vi "Firmware Manager.vi"(5 "Firmware Backup Folder":path, 6 "cRIO IP Address":string="172.16.0.2", 7 "Action":u8(ring) items=["Back Up Firmware to Files", "Update Firmware from Files"]) -> ()   [LabVIEW 2018]
doc: "Utility to save/restore/copy LabVIEW RT target configurations.\nUsage:\n rtcp [-c|-d] [-s] source destination\nwhere source, destination can be either IP address or folder path\nOptions: \ndefault (no option) - copy from target to target (using host's temporary folder):\n rtcp IPsource IPdestination\n-c - save an image of RT system in local folder:\n rtcp -c IPsource dst_folder\n-d - apply saved image or a patch to target:\n rtcp -d src_folder IPdestination\n-s - copy software only, skipping all other files (Installed Software Checkbox)"
uses:
  <vilib>/Utility/config.llb/Read Key (String).vi
  <vilib>/Utility/config.llb/NI_LVConfig.lvlib
panel:
  in  "Browse IP":bool
  out "Description":string
  in  "Exit":bool
  in  "Start Copying":bool
  out "Messages":string
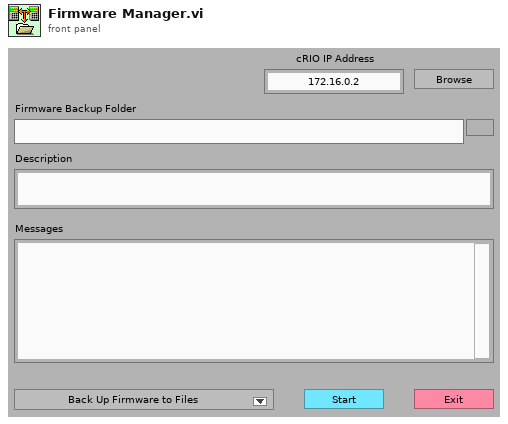
[diagram p1: front panel]
types:
  T1 = cluster{"Model":string, "MAC Address":string, "Hostname":string}
  T2 = typedef "NI_LVConfig.lvlib/Config Data RefNum.ctl" = refnum<k1>
  T3 = cluster{"cRIO IP Address":string, string, "Firmware Backup Folder":path, "Source":enum32{"RT Target", "Folder"}}
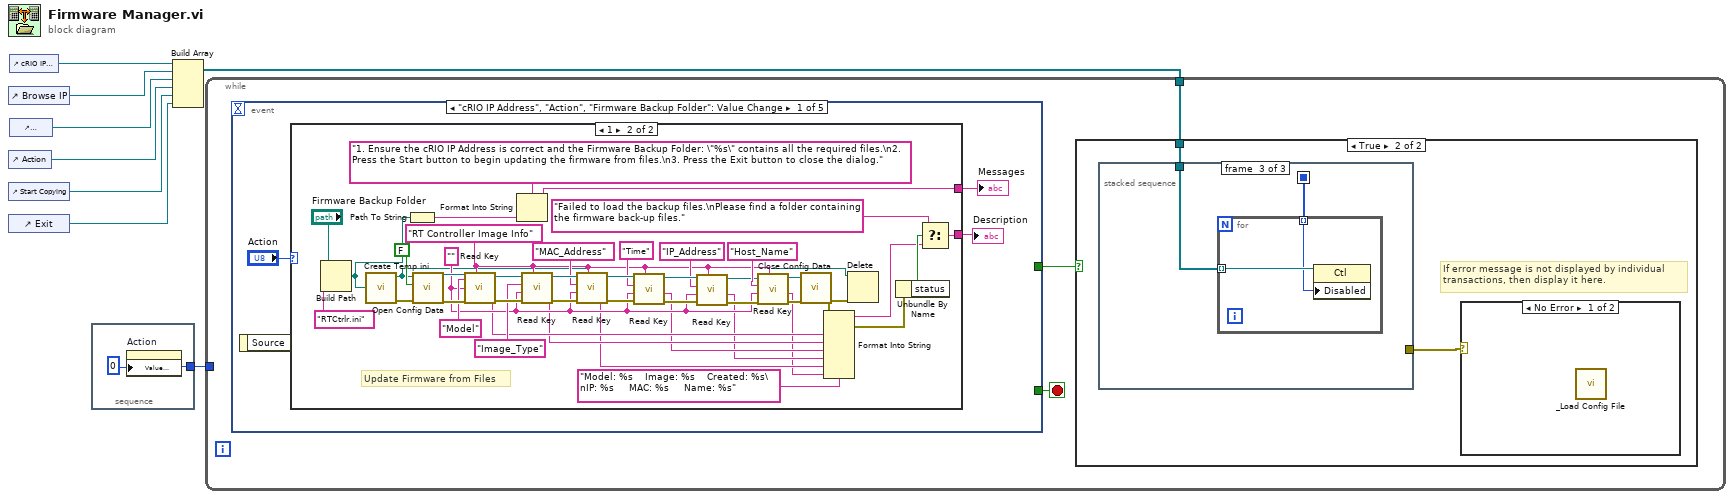
[diagram p0: block diagram]
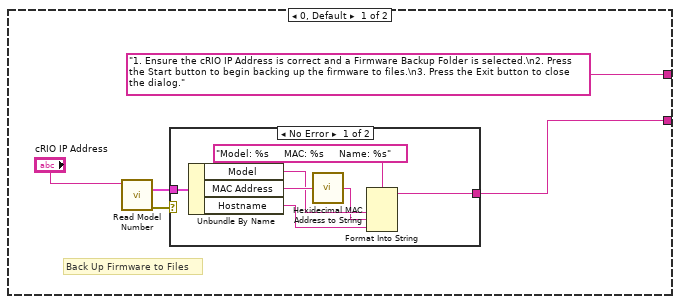
[diagram p2: hidden frame]
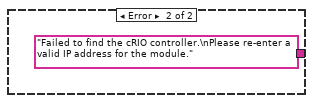
[diagram p3: hidden frame]
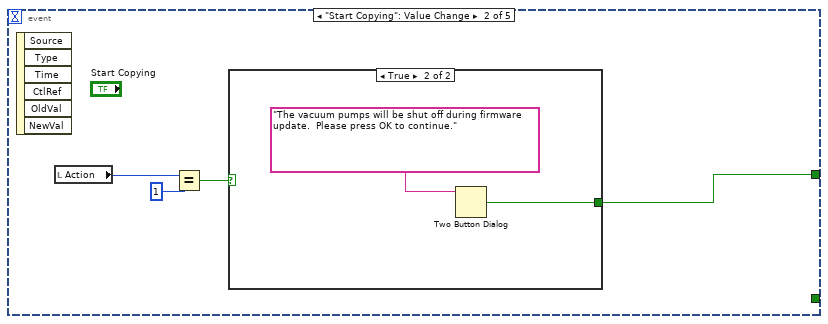
[diagram p4: hidden frame]
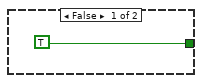
[diagram p5: hidden frame]
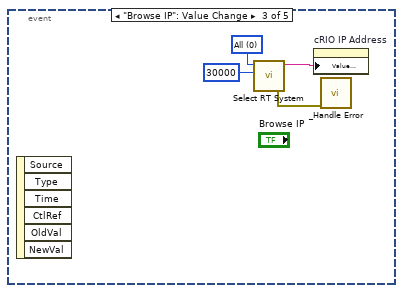
[diagram p6: hidden frame]
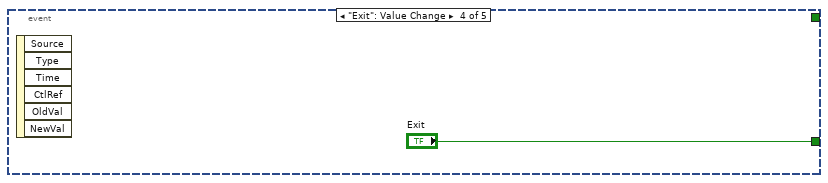
[diagram p7: hidden frame]
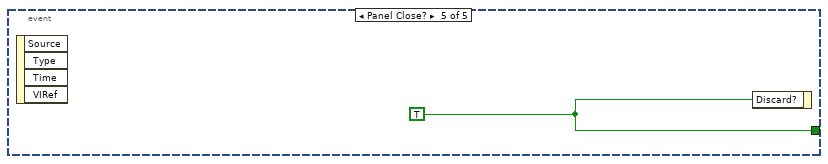
[diagram p8: hidden frame]
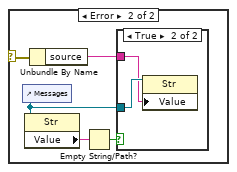
[diagram p10: hidden frame]
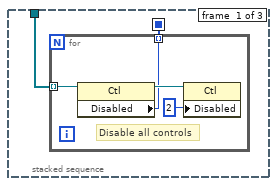
[diagram p12: hidden frame]
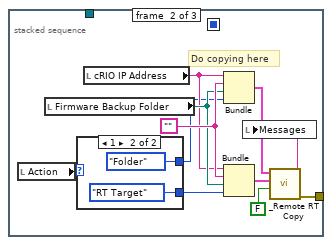
[diagram p13: hidden frame]
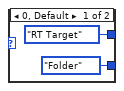
[diagram p14: hidden frame]
diagram:
  n1 = control-ref of="Browse IP"() -> (w7:refnum<vi>)
  n2 = control-ref of="Action"() -> (w5:refnum<vi>)
  n3 = control-ref of="Start Copying"() -> (w3:refnum<vi>)
  n4 = control-ref of="Exit"() -> (w2:refnum<vi>)
  n5 = control-ref of="cRIO IP Address"() -> (w8:refnum<vi>)
  n6 = control-ref of="Firmware Backup Folder"() -> (w6:refnum<vi>)
  n7 = stacked-sequence {
    tunnel: [w9] -> w1
    frame #0 {
      w9 = u8 0
      n8 = property on="Action" class="Ring (strict)"("Value (Signaling)"=w9) -> ()  [unwired: 2 in, 2 out]
    }
  }
  n9 = Build Array(w8, w7, w6, w5, w3, w2) -> (w4:refnum<vi>[])
  n10 = while {
    tunnel: w4 -> [w10]
    tunnel: w1 -> [_]
    stop <- w11 stop-if-true
    n11 = event shown="[0] \"cRIO IP Address\", \"Action\", \"Firmware Backup Folder\": Value Change" {
      selector: _ -> [_ _ _ _ _]
      dyn-events: _ -> [_ _ _ _ _]
      timeout: _ -> [_ _ _ _ _]
      tunnel: [_ _ _ "Exit" w85] -> w11
      tunnel: [_ w73 _ _ _] -> w12
      event "cRIO IP Address", "Action", "Firmware Backup Folder": Value Change {
        n12 = event-data() -> ()  [unwired: 2 out]
        n13 = case shown="1" "Action" {
          tunnel: [w18 w38] -> w15
          tunnel: ["1. Ensure the cRIO IP Address is correct and a Firmware Backup Folder is selected.\n2. Press the Start button to begin backing up the firmware to files.\n3. Press the Exit button to close the dialog." ("t") w34] -> w13
          frame 0, Default {
            # "Back Up Firmware to Files"
            n14 = call "Read Model Number.vi"("String"="cRIO IP Address") -> ("error out"=w19:errorcluster, "Target Info"=w20:T1)  [unwired: 9 in]
            n15 = case shown="No Error" w19 {
              tunnel: w20 -> [w27 _]
              tunnel: [w21 "Failed to find the cRIO controller.\nPlease re-enter a valid IP address for the module." ("t")] -> w18
              frame No Error {
                n16 = Unbundle By Name(w27) -> ("Model"=w24:string, "MAC Address"=w26:string, "Hostname"=w22:string)
                n17 = call <userlib>:"Hexidecimal MAC Address to String.vi"("MAC Address"=w26) -> ("MAC Address ("=w23:string)
                n18 = Format Into String(format string="Model: %s     MAC: %s     Name: %s", w24, w23, w22) -> (resulting string=w21:string)  [unwired: 2 in, 1 out]
              }
              frame Error {
              }
            }
          }
          frame 1 {
            w47 = ""
            w36 = "RT Controller Image Info" ("section")
            # "Update Firmware from Files"
            n19 = Build Path(base path="Firmware Backup Folder", name or relative path="RTCtrlr.ini") -> (appended path=w32:path)
            n20 = call "Create Temp ini.vi"("Original ini path"=w32) -> ("error out"=w31:errorcluster, "Temp ini path"=w29:path)  [unwired: 9 in]
            n21 = Path To String(path=w32) -> (string=w35:string)
            n22 = call <vilib>:"Open Config Data.vi"("error in (no error)"=w31, "create file if necessary (T)"=FALSE ("create file if necessary? (T)"), "configuration file path"=w29) -> ("error out"=w70:errorcluster, "refnum"=w71:T2)  [unwired: 6 in, 1 out]
            n23 = call-poly <vilib>:"Read Key.vi"("section"=w36, "error in (no error)"=w70, "default value"=w47, "key"="Model", "refnum"=w71) -> ("error out"=w67:errorcluster, "value"=w45:string, "refnum out"=w68:T2)  [unwired: 1 in, 3 out]
            n24 = Format Into String(format string="1. Ensure the cRIO IP Address is correct and the Firmware Backup Folder: \"%s\" contains all the required files.\n2. Press the Start button to begin updating the firmware from files.\n3. Press the Exit button to close the dialog." ("t"), w35) -> (resulting string=w34:string)  [unwired: 2 in, 1 out]
            n25 = call-poly <vilib>:"Read Key.vi"("section"=w36, "error in (no error)"=w67, "default value"=w47, "key"="Image_Type", "refnum"=w68) -> ("error out"=w64:errorcluster, "value"=w44:string, "refnum out"=w65:T2)  [unwired: 1 in, 3 out]
            n26 = call-poly <vilib>:"Read Key.vi"("section"=w36, "error in (no error)"=w64, "default value"=w47, "key"="MAC_Address", "refnum"=w65) -> ("error out"=w60:errorcluster, "value"=w41:string, "refnum out"=w61:T2)  [unwired: 1 in, 3 out]
            n27 = call-poly <vilib>:"Read Key.vi"("section"=w36, "error in (no error)"=w60, "default value"=w47, "key"="Time", "refnum"=w61) -> ("error out"=w50:errorcluster, "value"=w43:string, "refnum out"=w51:T2)  [unwired: 1 in, 3 out]
            n28 = call-poly <vilib>:"Read Key.vi"("section"=w36, "error in (no error)"=w50, "default value"=w47, "key"="IP_Address", "refnum"=w51) -> ("error out"=w48:errorcluster, "value"=w42:string, "refnum out"=w49:T2)  [unwired: 1 in, 3 out]
            n29 = call-poly <vilib>:"Read Key.vi"("section"=w36, "error in (no error)"=w48, "default value"=w47, "key"="Host_Name", "refnum"=w49) -> ("error out"=w58:errorcluster, "value"=w40:string, "refnum out"=w59:T2)  [unwired: 1 in, 3 out]
            n30 = call <vilib>:"Close Config Data.vi"("error in (no error)"=w58, "refnum"=w59) -> ("error out"=w30:errorcluster)  [unwired: 1 in, 8 out]
            n31 = Format Into String(format string="Model: %s    Image: %s    Created: %s\nIP: %s     MAC: %s     Name: %s", error in=w30, w45, w44, w43, w42, w41, w40) -> (resulting string=w53:string, error out=w55:errorcluster)  [unwired: 1 in]
            n32 = Delete(path (use dialog)=w29, error in=w30) -> ()  [unwired: 3 in, 3 out]
            n33 = Unbundle By Name(w55) -> ("status"=w54:bool)
            n34 = Select(t="Failed to load the backup files.\nPlease find a folder containing the firmware back-up files.", s=w54, f=w53) -> (s? t:f=w38:string)
          }
        }
        "Description" <- w15
        "Messages" <- w13
      }
      event "Start Copying": Value Change {
        n35 = event-data() -> ()  [unwired: 7 out]
        n36 = local read "Action"() -> (w76:u8)
        n37 = Equal?(x=w76, y=u8 1) -> (x = y?=w74:bool)
        n38 = case shown="True" w74 {
          tunnel: [TRUE w78] -> w73
          frame False {
          }
          frame True {
            n39 = Two Button Dialog(message="The vacuum pumps will be shut off during firmware update.  Please press OK to continue.") -> (T button?=w78:bool)  [unwired: 2 out]
          }
        }
      }
      event "Browse IP": Value Change {
        w83 = u16 0 items=["All", "Configured only", "Unconfigured only"] ("Display Mode")
        n40 = event-data() -> ()  [unwired: 7 out]
        n41 = call "Select RT System.vi"("Timeout ms (4000)"=30000, "Display Mode"=w83) -> ("error out"=w80:errorcluster, "IP Addresst Out"=w81:string)  [unwired: 1 in, 3 out]
        n42 = property on="cRIO IP Address" class="Str"("Value (Signaling)"=w81) -> ()  [unwired: 2 in, 2 out]
        n43 = call "_Handle Error.vi"("error in (no error)"=w80) -> ()  [unwired: 2 in, 5 out]
      }
      event "Exit": Value Change {
        n44 = event-data() -> ()  [unwired: 7 out]
      }
      event Panel Close? {
        w85 = TRUE ("Exit 2")
        n45 = event-data() -> ()  [unwired: 5 out]
        n46 = event-data("Discard?"=w85) -> ()  [unwired: 1 in, 1 out]
      }
    }
    n47 = case shown="True" w12 {
      tunnel: w10 -> [_ w87]
      frame False {
      }
      frame True {
        # "If error message is not displayed by individual \ntransactions, then display it here."
        n48 = stacked-sequence {
          seq-local: [w95 _ _] -> [_ _ w116]
          tunnel: w87 -> [w96 _ w117]
          tunnel: [_ w109 _] -> w86
          frame #0 {
            n49 = for {
              tunnel: w96 -> [w99] mode=indexing
              tunnel: [w97] -> w95 mode=indexing
              # "Disable all controls"
              n50 = property class="Ctl"(reference=w99) -> (reference out=w98:refnum<vi>, "Disabled"=w97:u8)  [unwired: 1 in, 1 out]
              n51 = property class="Ctl"(reference=w98, "Disabled"=u8 2) -> ()  [unwired: 1 in, 2 out]
            }
          }
          frame #1 {
            w107 = ""
            # "Do copying here"
            n52 = local read "Action"() -> (w104:u8)
            n53 = local read "Firmware Backup Folder"() -> (w106:path)
            n54 = case shown="1" w104 {
              tunnel: [enum32{"RT Target", "Folder"}."RT Target" ("Source") enum32{"RT Target", "Folder"}."Folder" ("Source")] -> w102
              tunnel: [enum32{"RT Target", "Folder"}."Folder" ("Source") enum32{"RT Target", "Folder"}."RT Target" ("Source")] -> w103
              frame 0, Default {
              }
              frame 1 {
              }
            }
            n55 = local read "cRIO IP Address"() -> (w105:string)
            n56 = Bundle("cRIO IP Address"=w105, w107, "Firmware Backup Folder"=w106, "Source"=w102) -> (w110:T3)  [unwired: 1 out]
            n57 = Bundle("cRIO IP Address"=w105, w107, "Firmware Backup Folder"=w106, "Source"=w103) -> (w111:T3)  [unwired: 1 out]
            n58 = call "_Remote RT Copy.vi"("Copy software only"=FALSE, "Image Destination"=w111, "Image Source"=w110) -> ("Error Out"=w109:errorcluster, "Messages"=w101:string)  [unwired: 1 in, 4 out]
            n59 = local write "Messages"(w101) -> ()
          }
          frame #2 {
            n60 = for {
              tunnel: w117 -> [w119] mode=indexing
              tunnel: w116 -> [w118] mode=indexing
              n61 = property class="Ctl"(reference=w119, "Disabled"=w118) -> ()  [unwired: 1 in, 2 out]
            }
          }
        }
        n62 = case shown="No Error" w86 {
          selector: w86 -> [_ w88]
          frame No Error {
            n63 = call "_Load Config File.vi"() -> ()  [unwired: 2 in, 2 out]
          }
          frame Error {
            n64 = control-ref of="Messages"() -> (w90:refnum<vi>)
            n65 = property class="Str"(reference=w90) -> ("Value"=w92:string)  [unwired: 1 in, 2 out]
            n66 = Unbundle By Name(w88) -> ("source"=w89:string)
            n67 = Empty String/Path?(string/path=w92) -> (empty?=w91:bool)
            n68 = case shown="True" w91 {
              tunnel: w90 -> [_ w94]
              tunnel: w89 -> [_ w93]
              frame False {
              }
              frame True {
                n69 = property class="Str"(reference=w94, "Value"=w93) -> ()  [unwired: 1 in, 2 out]
              }
            }
          }
        }
      }
    }
  }
